vi "Do.vi"(8 "error in (no error)":errorcluster, 11 "Engine in":refnum<class "Engine.lvclass">) -> (0 "error out":errorcluster, 3 "Engine out":refnum<class "Engine.lvclass">)   [LabVIEW 2019, in "RT_Game.lvlib" / "Engine.lvclass"]
uses:
  Engine.lvclass
  Engine.lvclass/Engine.ctl
  Game/Game.lvclass/Game.ctl
  Game/Read SwitchGame.vi
  Game/Game.lvclass
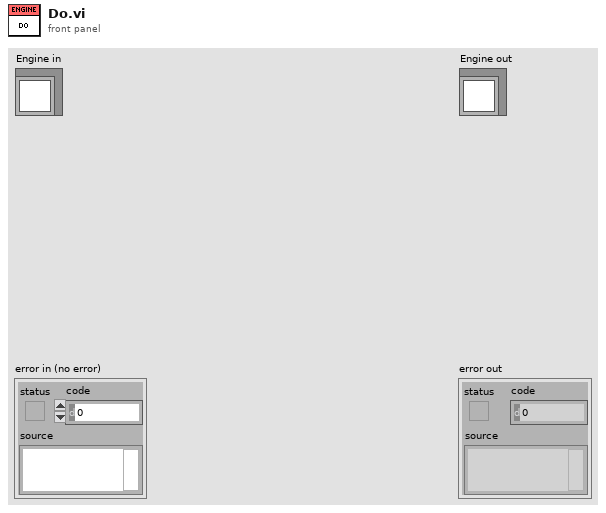
[diagram p1: front panel]
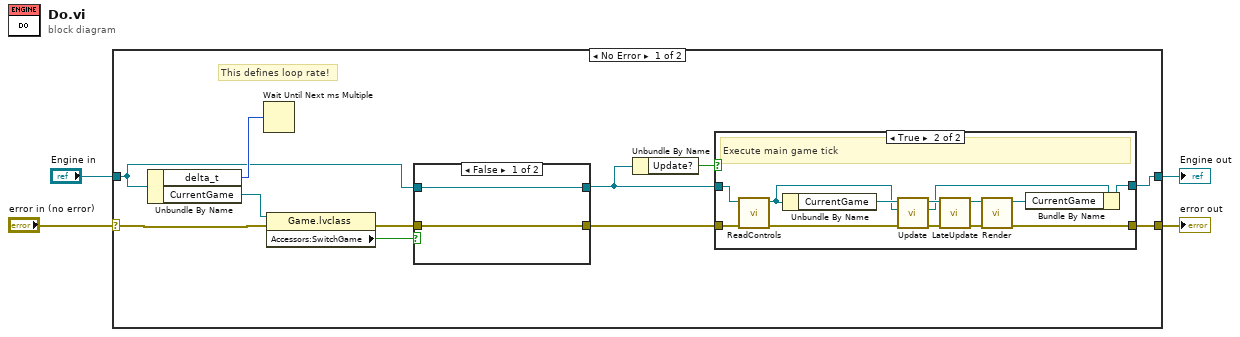
[diagram p0: block diagram]
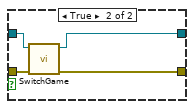
[diagram p2: hidden frame]
diagram:
  n1 = case shown="No Error" "error in (no error)" {
    selector: "error in (no error)" -> [w9 w38]
    tunnel: [w15 w38] -> w3
    tunnel: [w7 w37] -> w1
    tunnel: "Engine in" -> [w8 w37]
    frame No Error {
      # "This defines loop rate!"
      n2 = Unbundle By Name(w8) -> ("delta_t"=w10:u16, "CurrentGame"=w13:refnum<class "Game.lvclass">)
      n3 = Wait Until Next ms Multiple(millisecond multiple=w10) -> ()  [unwired: 1 out]
      n4 = property class="Game.lvclass"(reference=w13, error in=w9) -> (error out=w14:errorcluster, "Accessors:SwitchGame"=w11:bool)  [unwired: 1 out]
      n5 = case shown="False" w11 {
        tunnel: w14 -> [w16 w21]
        tunnel: [w16 w20] -> w12
        tunnel: w8 -> [w17 w18]
        tunnel: [w17 w19] -> w6
        frame False {
        }
        frame True {
          n6 = call "SwitchGame.vi"("error in (no error)"=w21, "Engine in"=w18) -> ("error out"=w20:errorcluster, "Engine out"=w19:refnum<class "Engine.lvclass">)  [unwired: 8 in]
        }
      }
      n7 = Unbundle By Name(w6) -> ("Update?"=w5:bool)
      n8 = case shown="True" w5 {
        tunnel: w12 -> [w23 w36]
        tunnel: [w23 w34] -> w15
        tunnel: w6 -> [w22 w26]
        tunnel: [w22 w30] -> w7
        frame False {
        }
        frame True {
          # "Execute main game tick"
          n9 = call "ReadControls.vi"("error in (no error)"=w36, "Engine in"=w26) -> ("error out"=w27:errorcluster, "Engine out"=w25:refnum<class "Engine.lvclass">)  [unwired: 8 in]
          n10 = Unbundle By Name(w25) -> ("CurrentGame"=w28:refnum<class "Game.lvclass">)
          n11 = call-dynamic "Update.vi"("error in (no error)"=w27, "Engine in"=w25, "Game in"=w28) -> ("error out"=w35:errorcluster, "Engine out"=w24:refnum<class "Engine.lvclass">, "Game out"=w32:refnum<class "Game.lvclass">)  [unwired: 6 in]
          n12 = call-dynamic "LateUpdate.vi"("error in (no error)"=w35, "Game in"=w32) -> ("error out"=w33:errorcluster, "Game out"=w31:refnum<class "Game.lvclass">)  [unwired: 8 in]
          n13 = call-dynamic "Render.vi"("error in (no error)"=w33, "Game in"=w31) -> ("error out"=w34:errorcluster, "Game out"=w29:refnum<class "Game.lvclass">)  [unwired: 8 in]
          n14 = Bundle By Name(cluster=w24, "CurrentGame"=w29) -> (w30:refnum<class "Engine.lvclass">)
        }
      }
    }
    frame Error {
    }
  }
  "error out" <- w3
  "Engine out" <- w1
